vi "Write ErrorColorText.vi"(8 "error in (no error)":errorcluster, 10 "CorrectColorBG":u32(colorbox), 11 "PhoneFromField in":refnum<class "PhoneFromField.lvclass">) -> (0 "error out":errorcluster, 3 "PhoneFromField out":refnum<class "PhoneFromField.lvclass">)   [LabVIEW 2019, in "PhoneFromField.lvclass"]
uses:
  PhoneFromField.lvclass
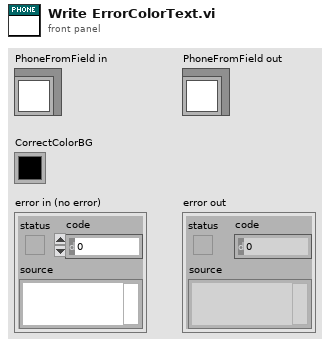
[diagram p1: front panel]
types:
  T1 = typedef "PhoneFromField.lvclass/State Data.ctl" = cluster{"CorrectColorBG":u32}
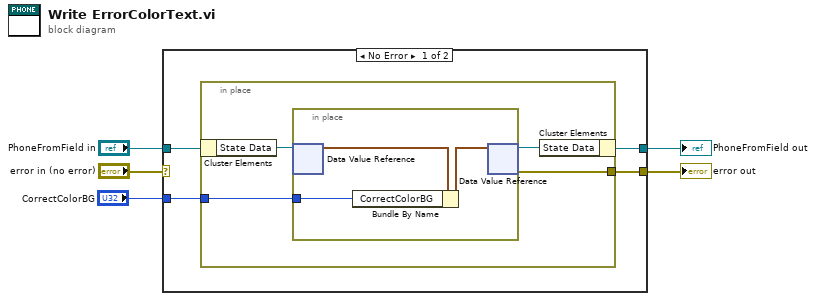
[diagram p0: block diagram]
diagram:
  n1 = case shown="No Error" "error in (no error)" {
    selector: "error in (no error)" -> [_ w18]
    tunnel: [w6 w18] -> w4
    tunnel: [w7 w17] -> w2
    tunnel: "PhoneFromField in" -> [w9 w17]
    tunnel: "CorrectColorBG" -> [w8 _]
    frame No Error {
      n2 = in-place {
        in-place-border: w8 -> [w12]
        in-place-border: [w10] -> w6
        n3 = in-place-cluster #1(w9) -> ("State Data"=w13:refnum<data-value>)
        n4 = in-place {
          in-place-border: w12 -> [w15]
          n5 = in-place-dvr #2(w13) -> (w16:T1)  [unwired: 1 out]
          n6 = Bundle By Name(cluster=w16, "CorrectColorBG"=w15) -> (w14:T1)
          n7 = in-place-dvr #2(w14) -> (w11:refnum<data-value>, w10:errorcluster)
        }
        n8 = in-place-cluster #1("State Data"=w11) -> (w7:refnum<class "PhoneFromField.lvclass">)
      }
    }
    frame Error {
    }
  }
  "error out" <- w4
  "PhoneFromField out" <- w2
